vi "TPM with correction version 10-3-compare-1 scale factor_descan_20191023.vi"() -> ()   [LabVIEW 2018]
uses:
  Casao LabVIEW SDK 1.0.5/Haso/Data Haso/Wavefront parameters.ctl
  Casao LabVIEW SDK 1.0.5/Casao/Casao/Loop prefs.ctl
  Casao LabVIEW SDK 1.0.5/Haso/Data Haso/DataHaso.ctl
  <vilib>/Utility/file.llb/Read From Spreadsheet File (DBL).vi
  <vilib>/Utility/file.llb/Write To Spreadsheet File (DBL).vi
panel:
  out "error out 4":errorcluster
  out "error out 3":errorcluster
  out "error out 2":errorcluster
  out "error out":errorcluster
  in  "Descan  Rescan":bool
  in  "Camera              WF sensor":bool
  in  "Scale factor":dbl=1.0
  out "output path":path
  out "Model Coefficients (µm) after":sgl[](array[numeric])
  out "Model Coefficients (µm) before":sgl[](array[numeric])
  in  "stop":bool
  out "Slice now":dbl
  in  "Iteration #":u16(ring)=1 items=["1"=1, "2"=2, "3"=3, "4"=4, "5"=5]
  in  "AoExp Time":dbl(ring)=0.5 items=["0.2s"=0.2, "0.5s"=0.5, "1.0s"=1.0, "1.5s"=1.5]
  out "after correction":T1
  in  "Filter y tilt":bool=TRUE
  in  "Filter x tilt":bool=TRUE
  in  "Curvature filter":bool=TRUE
  out "PV":dbl
  out "RMS":dbl
  in  "Matrix path":path=path "D:/SystemAlignment/20191015_PathCheck_WFSalign/commandMatrix.aomc"
  in  "Offset path":path=path "D:/Data/100nm correction.dat"
  out "Camera image":u32[][](graph)
  out "RMS":dbl
  out "PV":dbl
  out "before correction":T1
  in  "Curvature filter":bool=TRUE
  in  "Filter y tilt":bool=TRUE
  in  "Filter x tilt":bool=TRUE
  out "after correction":dbl[][](graph) caption="Wavefront"
  out "before correction":dbl[][](graph) caption="Wavefront"
  in  "ImExp Time (s)":dbl(ring)=0.5 items=["0.2"=0.2, "0.5"=0.5, "1.0"=1.0, "4.0"=4.0, "8.0"=8.0]
  in  "Step size(um)":dbl
  in  "Laser Power%(0-100)":dbl=50.0
  in  "Slices #":dbl=2.0
  in  "Average Frame #":dbl=2.0
  in  "Correction":bool
  # "OFF"
  # "ON"
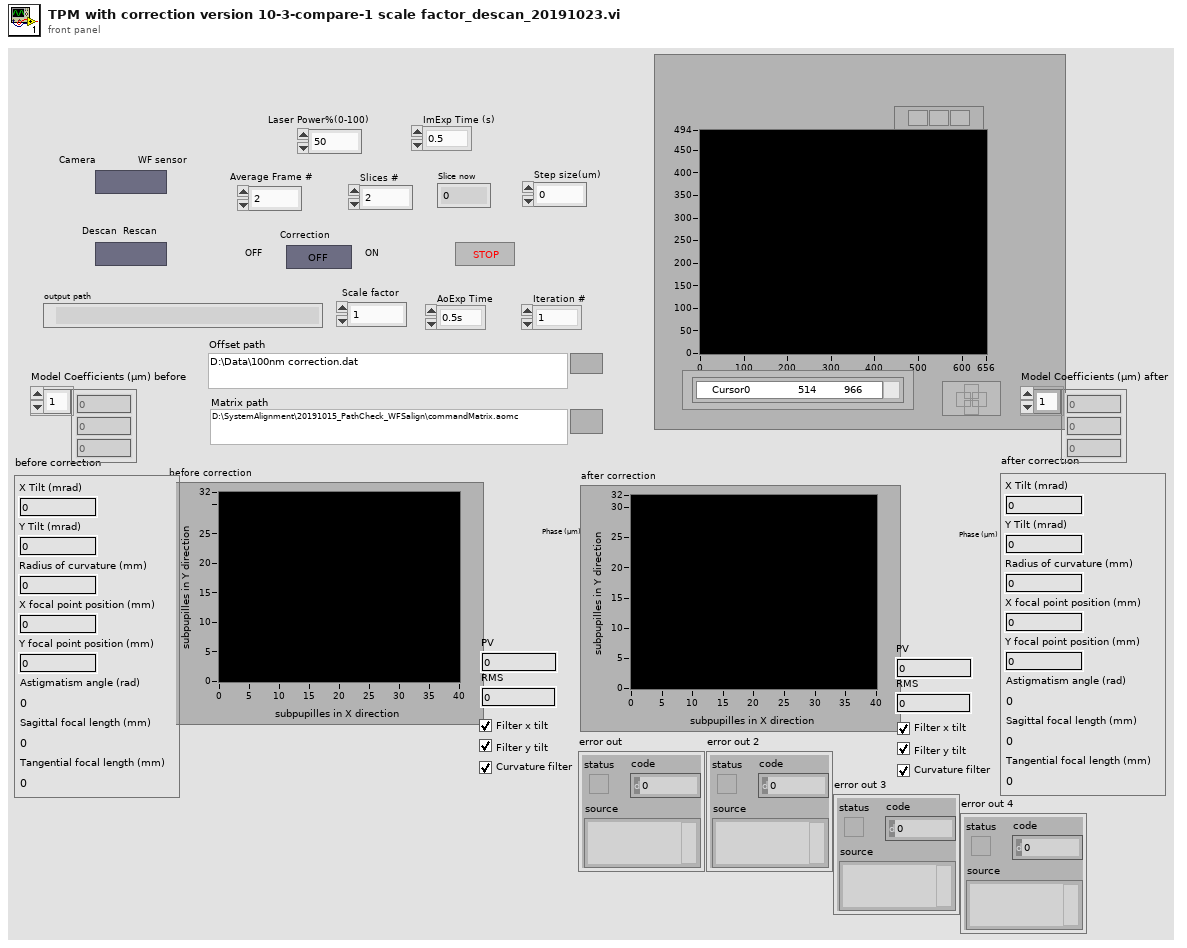
[diagram p1: front panel]
types:
  T1 = typedef "Wavefront parameters.ctl" = cluster{"X Tilt (mrad)":sgl, "Y Tilt (mrad)":sgl, "Radius of curvature (mm)":sgl, "X focal point position (mm)":sgl, "Y focal point position (mm)":sgl, "Astigmatism angle (rad)":sgl, "Sagittal focal length (mm)":sgl, "Tangential focal length (mm)":sgl}
  T2 = typedef "Loop prefs.ctl" = cluster{"Filter tilt on measurement (closed loop)":bool, "Correction gain (closed loop)":sgl, "Limit of subapertures off in CGP (%)":sgl, "Limit of saturated actuators (%)":sgl}
  T3 = cluster{"Filtre tilt X":bool, "Filtre tilt Y":bool, "Filtre courbure":bool}
  T4 = typedef "DataHaso.ctl" = i32
  T5 = cluster{"Measurement":T4, "Target":T4, "Manual target":T4}
  T6 = cluster{"Target for tilt":T4, "Target for focus":T4, "Target for all other aberrations":T4}
  T7 = typedef "Camera.ctl" = i32
  T8 = typedef "PhaseModul.ctl" = i32
  T9 = typedef "Haso.ctl" = i32
  T10 = typedef "Casao.ctl" = i32
  T11 = typedef "Image Compat.ctl" = cluster{"Signed/unsigned":bool, "Number of bits":T12, "Internal object id":i32, "Internal data id":i32}
  T12 = typedef "Data alignment enum.ctl" = enum16{"8", "16", "32"}
  T13 = typedef "Reconstruction prefs.ctl" = cluster{"Reconstruction type":enum16{"Modal", "Zonal"}, "Polynomial type":enum16{"Zernike", "Legendre"}, "Modal reconstruction prefs":T14, "Zonal reconstruction prefs":T17}
  T14 = typedef "Modal reconstruction prefs.ctl" = cluster{"Number of coefficients":u32, "Filtered coefficients":u32[], "RMS Zernike normalization":bool, "Matrix inversion method":u16, "Add zonal residual to modal fit ":bool, "Detection prefs":T15}
  T15 = typedef "PupilDetectionPrefs.ctl" = cluster{"Automatic pupil detection":bool, "Central occultation pupil":bool, "Semi-automatic pupil detection (find radius)":bool, "Semi-automatic pupil detection (find center)":bool, "Automatic pupil detection mode":enum16{"Contained", "Containing"}, "Start coordinates":cluster{"Pupil center (Zernike)":T16, "Pupil radius (Zernike)":sgl, "Pupil center (Legendre)":T16, "Pupil halfsize (Legendre)":T16}}
  T16 = typedef "Point2Df.ctl" = cluster{"X":sgl, "Y":sgl}
  T17 = typedef "Zonal reconstruction prefs.ctl" = cluster{"Number of weak iterations":u16, "Number of max iterations":u32, "Residual limit":sgl}
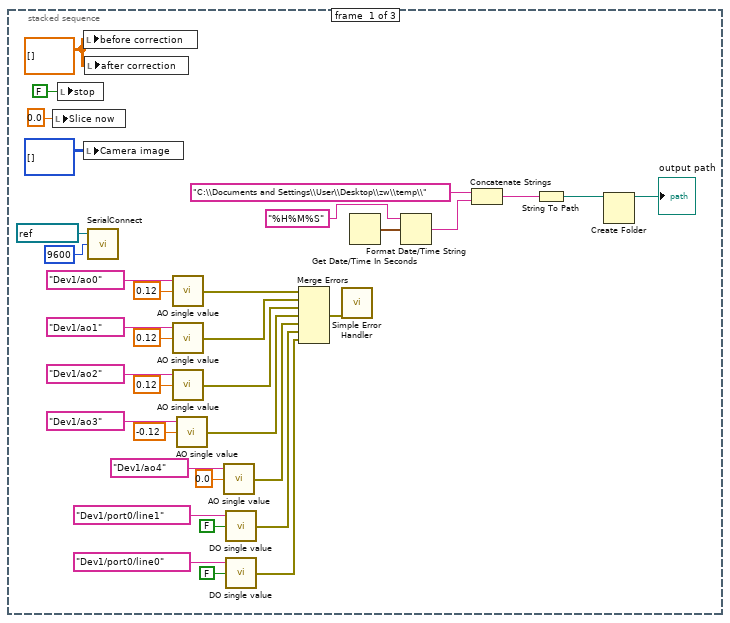
[diagram p2: hidden frame]
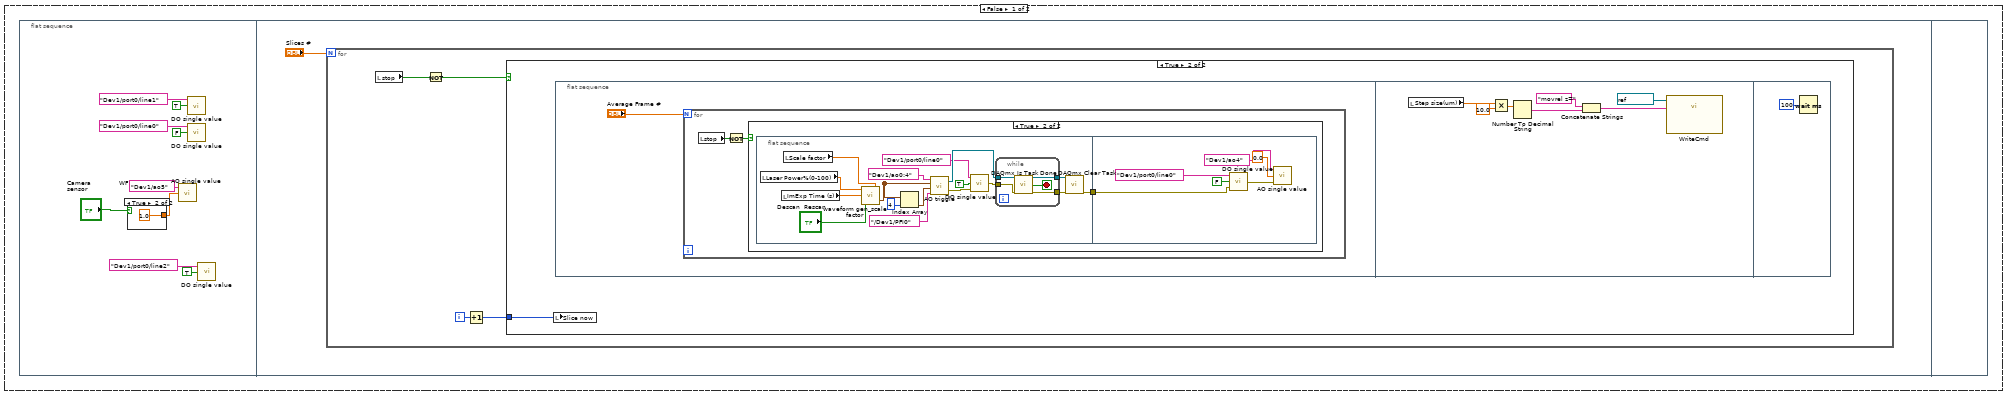
[diagram p3: hidden frame]
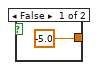
[diagram p4: hidden frame]
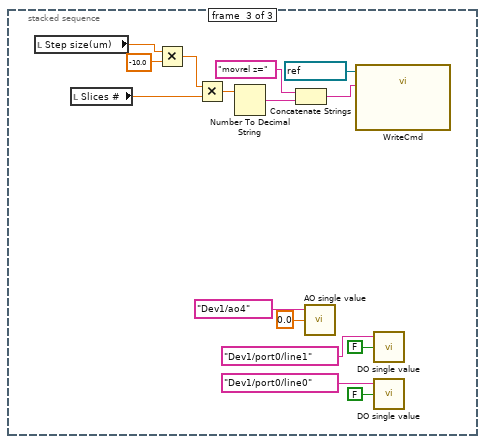
[diagram p12: hidden frame]
diagram:
  n1 = stacked-sequence {
    frame #0 {
      w34 = dbl[][] [] ("before correction")
      n2 = local write "Slice now"(0.0 ("Slice now")) -> ()
      n3 = local write "stop"(FALSE ("stop")) -> ()
      n4 = local write "before correction"(w34) -> ()
      n5 = local write "Camera image"(u32[][] [] ("Camera image")) -> ()
      n6 = local write "after correction"(w34) -> ()
      n7 = call "SerialConnect.vi"("baud rate (9600)"=u32 9600, "VISA resource name"=refnum<visa-resource-name> "COM1") -> ()  [unwired: 1 in, 3 out]
      n8 = call "AO single value.vi"("data"=0.12, "physical channels"=tag "Dev1/ao0") -> ("error out"=w17:errorcluster)  [unwired: 1 in]
      n9 = call "AO single value.vi"("data"=0.12, "physical channels"=tag "Dev1/ao1") -> ("error out"=w16:errorcluster)  [unwired: 1 in]
      n10 = call "AO single value.vi"("data"=0.12, "physical channels"=tag "Dev1/ao2") -> ("error out"=w15:errorcluster)  [unwired: 1 in]
      n11 = call "AO single value.vi"("data"=-0.12, "physical channels"=tag "Dev1/ao3") -> ("error out"=w14:errorcluster)  [unwired: 1 in]
      n12 = call "AO single value.vi"("data"=0.0, "physical channels"=tag "Dev1/ao4") -> ("error out"=w13:errorcluster)  [unwired: 1 in]
      n13 = call "DO single value.vi"("data"=FALSE, "lines"=tag "Dev1/port0/line1") -> ("error out"=w12:errorcluster)  [unwired: 1 in]
      n14 = call "DO single value.vi"("data"=FALSE, "lines"=tag "Dev1/port0/line0") -> ("error out"=w10:errorcluster)  [unwired: 1 in]
      n15 = Merge Errors(w17, w16, w15, w14, w13, w12, w10) -> (w11:errorcluster)
      n16 = call <vilib>:"Simple Error Handler.vi"("error in (no error)"=w11) -> ()  [unwired: 4 in, 5 out]
      n17 = Get Date/Time In Seconds() -> (seconds since 1Jan1904=w7:timestamp)
      n18 = Format Date/Time String(time format string (%c)="%H%M%S", seconds (now)=w7) -> (date/time string=w4:string)  [unwired: 1 in]
      n19 = Concatenate Strings("C:\\Documents and Settings\\User\\Desktop\\zw\\temp\\" ("string"), w4) -> (w3:string)
      n20 = String To Path(string=w3) -> (path=w2:path)
      n21 = Create Folder(path (use dialog)=w2) -> (created path=→"output path":path)  [unwired: 2 in, 2 out]
    }
    frame #1 {
      n22 = case shown="True" "Correction" {
        frame False {
          n23 = flat-sequence {
            frame #0 {
              n24 = case shown="True" "Camera              WF sensor" {
                tunnel: [-5.0 ("data") 1.0 ("data")] -> w40
                frame False {
                }
                frame True {
                }
              }
              n25 = call "AO single value.vi"("data"=w40, "physical channels"=tag "Dev1/ao5") -> ()  [unwired: 1 in, 1 out]
              n26 = call "DO single value.vi"("data"=TRUE, "lines"=tag "Dev1/port0/line1") -> ()  [unwired: 1 in, 1 out]
              n27 = call "DO single value.vi"("data"=FALSE, "lines"=tag "Dev1/port0/line0") -> ()  [unwired: 1 in, 1 out]
              n28 = call "DO single value.vi"("data"=TRUE, "lines"=tag "Dev1/port0/line2") -> ()  [unwired: 1 in, 1 out]
            }
            frame #1 {
              n29 = for {
                N: "Slices #" -> [_]
                i -> [w52]
                n30 = local read "stop"() -> (w50:bool)
                n31 = Not(x=w50) -> (.not. x?=w49:bool)
                n32 = Increment(x=w52) -> (x+1=w51:i32)
                n33 = case shown="True" w49 {
                  tunnel: w51 -> [_ w53]
                  frame False {
                  }
                  frame True {
                    n34 = local write "Slice now"(w53) -> ()
                    n35 = flat-sequence {
                      frame #0 {
                        n36 = for {
                          N: "Average Frame #" -> [_]
                          n37 = local read "stop"() -> (w55:bool)
                          n38 = Not(x=w55) -> (.not. x?=w56:bool)
                          n39 = case shown="True" w56 {
                            frame False {
                            }
                            frame True {
                              n40 = flat-sequence {
                                tunnel: [w63] -> w57
                                tunnel: w57 -> [w81]
                                frame #0 {
                                n41 = local read "Laser Power%(0-100)"() -> (w60:dbl)
                                n42 = local read "ImExp Time (s)"() -> (w61:dbl)
                                n43 = local read "Scale factor"() -> (w59:dbl)
                                n44 = call "waveform gen_scale factor.vi"("Scale factor"=w59, "Boolean"="Descan  Rescan", "Exposure Time (s)"=w61, "Laser Power%(0-100)"=w60) -> ("waveform"=w62:waveform(dbl)[])
                                n45 = Index Array(array=w62, index=4) -> (element=w71:waveform(dbl))
                                n46 = call "AO triggle.vi"("physical channels"=tag "Dev1/ao0:4", "data"=w62, "waveform"=w71, "trig source"=tag "/Dev1/PFI0") -> ("task out"=w68:refnum<k21>, "error out"=w65:errorcluster)  [unwired: 1 in]
                                n47 = call "DO single value.vi"("error in"=w65, "data"=TRUE, "lines"=tag "Dev1/port0/line0") -> ("error out"=w64:errorcluster)
                                n48 = while {
                                tunnel: [w79] -> w74
                                tunnel: [w78] -> w73
                                tunnel: w68 -> [w76]
                                tunnel: w64 -> [w75]
                                stop <- w77 stop-if-true
                                n49 = call <vilib>:"DAQmx Is Task Done.vi"("task/channels in"=w76, "error in"=w75) -> ("task out"=w79:refnum<k21>, "task done?"=w77:bool, "error out"=w78:errorcluster)  [unwired: 11 in]
                                }
                                n50 = call <vilib>:"DAQmx Clear Task.vi"("task in"=w74, "error in"=w73) -> ("error out"=w63:errorcluster)  [unwired: 13 in]
                                }
                                frame #1 {
                                n51 = call "DO single value.vi"("error in"=w81, "data"=FALSE, "lines"=tag "Dev1/port0/line0") -> ("error out"=w80:errorcluster)
                                n52 = call "AO single value.vi"("error in"=w80, "data"=0.0, "physical channels"=tag "Dev1/ao4") -> ()  [unwired: 1 out]
                                }
                              }
                            }
                          }
                        }
                      }
                      frame #1 {
                        n53 = local read "Step size(um)"() -> (w86:dbl)
                        n54 = Multiply(x=w86, y=10.0) -> (x*y=w88:dbl)
                        n55 = Number To Decimal String(number=w88) -> (decimal integer string=w91:string)  [unwired: 1 in]
                        n56 = Concatenate Strings("movrel z=", w91) -> (w90:string)
                        n57 = call "WriteCmd.vi"("Command"=w90, "VISA resource name"=refnum<visa-resource-name> "COM1") -> ()  [unwired: 1 in, 1 out]
                      }
                      frame #2 {
                        n58 = Wait (ms)(milliseconds to wait=u32 100) -> ()  [unwired: 1 out]
                      }
                    }
                  }
                }
              }
            }
            frame #2 {
            }
          }
        }
        frame True {
          n59 = flat-sequence {
            tunnel: [w102] -> w101
            tunnel: [w111] -> w100
            tunnel: [w110] -> w99
            tunnel: [w102] -> w98
            tunnel: [w109] -> w97
            tunnel: [w108] -> w95
            tunnel: [w103] -> w94
            tunnel: w101 -> [w128]
            tunnel: w100 -> [w127]
            tunnel: w99 -> [w126]
            tunnel: w98 -> [w122]
            tunnel: w97 -> [w120]
            tunnel: [w125] -> w96
            tunnel: w95 -> [w124]
            tunnel: w94 -> [w118]
            tunnel: w96 -> [w655]
            frame #0 {
              n60 = call "AO single value.vi"("data"=0.0, "physical channels"=tag "Dev1/ao4") -> ()  [unwired: 1 in, 1 out]
              n61 = local read "AoExp Time"() -> (w112:dbl)
              n62 = call-poly <vilib>:"Read From Spreadsheet File.vi"("format (%.3f)"="%.8f", "file path (dialog if empty)"="Offset path") -> ("first row"=w103:dbl[])  [unwired: 5 in, 4 out]
              n63 = call "DO single value.vi"("data"=TRUE, "lines"=tag "Dev1/port0/line1") -> ()  [unwired: 1 in, 1 out]
              n64 = call "DO single value.vi"("data"=FALSE, "lines"=tag "Dev1/port0/line0") -> ()  [unwired: 1 in, 1 out]
              n65 = call "AO init.vi"("Exposure duration specified (s)"=w112, "Commands in"=w103, "Matrix path"="Matrix path") -> ("error out"=w102:errorcluster, "Camera"=w111:T7, "Mirror"=w108:T8, "Haso"=w110:T9, "Casao"=w109:T10)  [unwired: 3 in, 1 out]
              "error out" <- w102
            }
            frame #1 {
              n66 = local read "Slices #"() -> (w129:dbl)
              n67 = call "Casao Set Preferences.vi"("error in (no error)"=w122, "Loop preferences"=T2 {"Filter tilt on measurement (closed loop)"=FALSE, "Correction gain (closed loop)"=0.75, "Limit of subapertures off in CGP (%)"=0.0, "Limit of saturated actuators (%)"=0.0}, "Casao"=w120) -> ("error out"=w121:errorcluster, "Casao (dup)"=w119:T10)  [unwired: 3 in]
              n68 = for {
                N: w129 -> [_]
                tunnel: w128 -> [w145]
                tunnel: w127 -> [w144]
                tunnel: w126 -> [w143]
                tunnel: w121 -> [w131]
                tunnel: [w142] -> w125
                tunnel: w124 -> [w133]
                tunnel: w119 -> [w141]
                tunnel: w118 -> [w134]
                i -> [w137]
                n69 = local read "stop"() -> (w139:bool)
                n70 = call "PhaseModul apply command.vi"("error in (no error)"=w131, "Commands in"=w134, "Mirror"=w133) -> ("error out"=w130:errorcluster, "Mirror (dup)"=w132:T8)  [unwired: 2 in, 1 out]
                n71 = Increment(x=w137) -> (x+1=w140:i32)
                n72 = local write "Slice now"(w140) -> ()
                n73 = Not(x=w139) -> (.not. x?=w138:bool)
                n74 = case shown="True" w138 {
                  tunnel: w145 -> [_ w180]
                  tunnel: w144 -> [_ w179]
                  tunnel: w143 -> [_ w178]
                  tunnel: w130 -> [_ w177]
                  tunnel: [w146 w174] -> w142
                  tunnel: w132 -> [_ w176]
                  tunnel: w141 -> [w146 w175]
                  frame False {
                  }
                  frame True {
                    n75 = flat-sequence {
                      tunnel: w175 -> [w185]
                      tunnel: w176 -> [w186]
                      tunnel: w177 -> [w187]
                      tunnel: w178 -> [w188]
                      tunnel: w179 -> [w189]
                      tunnel: w180 -> [w190]
                      tunnel: [w190] -> w152
                      tunnel: [w189] -> w151
                      tunnel: [w188] -> w150
                      tunnel: [w187] -> w149
                      tunnel: [w186] -> w148
                      tunnel: [w185] -> w147
                      tunnel: [w226] -> w173
                      tunnel: [w225] -> w172
                      tunnel: [w224] -> w171
                      tunnel: [w219] -> w170
                      tunnel: [w220] -> w169
                      tunnel: [w221] -> w168
                      tunnel: w152 -> [w226]
                      tunnel: w151 -> [w225]
                      tunnel: w150 -> [w224]
                      tunnel: w149 -> [w220]
                      tunnel: w148 -> [w221]
                      tunnel: w147 -> [w219]
                      tunnel: w173 -> [w268]
                      tunnel: w172 -> [w267]
                      tunnel: w171 -> [w266]
                      tunnel: w170 -> [w265]
                      tunnel: w169 -> [w264]
                      tunnel: [w244] -> w167
                      tunnel: [w243] -> w166
                      tunnel: [w239] -> w165
                      tunnel: [w237] -> w164
                      tunnel: [w235] -> w163
                      tunnel: w168 -> [w230]
                      tunnel: [w229] -> w162
                      tunnel: [w227] -> w161
                      tunnel: w167 -> [w410]
                      tunnel: w166 -> [w409]
                      tunnel: w165 -> [w407]
                      tunnel: w164 -> [w406]
                      tunnel: w163 -> [w405]
                      tunnel: [w404] -> w160
                      tunnel: w162 -> [w403]
                      tunnel: [w402] -> w159
                      tunnel: [w401] -> w158
                      tunnel: [w400] -> w157
                      tunnel: [w399] -> w156
                      tunnel: [w398] -> w155
                      tunnel: w161 -> [w397]
                      tunnel: [w397] -> w154
                      tunnel: w160 -> [w617]
                      tunnel: [w617] -> w153
                      tunnel: w159 -> [w607]
                      tunnel: w158 -> [w606]
                      tunnel: w157 -> [w605]
                      tunnel: w156 -> [w595]
                      tunnel: w155 -> [w596]
                      tunnel: w154 -> [w594]
                      tunnel: w153 -> [w618]
                      tunnel: [w618] -> w174
                      frame #0 {
                        n76 = local read "Average Frame #"() -> (w184:dbl)
                        n77 = Wait (ms)(milliseconds to wait=u32 100) -> ()  [unwired: 1 out]
                        n78 = call "AO single value.vi"("data"=-5.0, "physical channels"=tag "Dev1/ao5") -> ()  [unwired: 1 in, 1 out]
                        n79 = for {
                          N: w184 -> [_]
                          n80 = local read "stop"() -> (w191:bool)
                          n81 = Not(x=w191) -> (.not. x?=w192:bool)
                          n82 = case shown="True" w192 {
                            frame False {
                            }
                            frame True {
                              n83 = flat-sequence {
                                frame #0 {
                                n84 = local read "Laser Power%(0-100)"() -> (w194:dbl)
                                n85 = local read "ImExp Time (s)"() -> (w195:dbl)
                                n86 = local read "Scale factor"() -> (w193:dbl)
                                n87 = call "waveform gen_scale factor.vi"("Scale factor"=w193, "Boolean"=TRUE, "Exposure Time (s)"=w195, "Laser Power%(0-100)"=w194) -> ("waveform"=w197:waveform(dbl)[])
                                n88 = Index Array(array=w197, index=4) -> (element=w205:waveform(dbl))
                                n89 = call "AO triggle.vi"("physical channels"=tag "Dev1/ao0:4", "data"=w197, "waveform"=w205, "trig source"=tag "/Dev1/PFI0") -> ("task out"=w202:refnum<k21>, "error out"=w199:errorcluster)  [unwired: 1 in]
                                n90 = call "DO single value.vi"("error in"=w199, "data"=TRUE, "lines"=tag "Dev1/port0/line0") -> ("error out"=w198:errorcluster)
                                n91 = while {
                                tunnel: [w213] -> w208
                                tunnel: [w212] -> w207
                                tunnel: w202 -> [w210]
                                tunnel: w198 -> [w209]
                                stop <- w211 stop-if-true
                                n92 = call <vilib>:"DAQmx Is Task Done.vi"("task/channels in"=w210, "error in"=w209) -> ("task out"=w213:refnum<k21>, "task done?"=w211:bool, "error out"=w212:errorcluster)  [unwired: 11 in]
                                }
                                n93 = call <vilib>:"DAQmx Clear Task.vi"("task in"=w208, "error in"=w207) -> ()  [unwired: 13 in, 1 out]
                                }
                                frame #1 {
                                n94 = call "AO single value.vi"("data"=0.0, "physical channels"=tag "Dev1/ao4") -> ()  [unwired: 1 in, 1 out]
                                n95 = call "DO single value.vi"("data"=FALSE, "lines"=tag "Dev1/port0/line0") -> ()  [unwired: 1 in, 1 out]
                                }
                              }
                            }
                          }
                        }
                      }
                      frame #1 {
                        n96 = call "AO single value.vi"("data"=1.0, "physical channels"=tag "Dev1/ao5") -> ("error out"=→"error out 4":errorcluster)  [unwired: 1 in]
                      }
                      frame #2 {
                        n97 = flat-sequence {
                          tunnel: [w277] -> w263
                          tunnel: [w276] -> w262
                          tunnel: [w275] -> w261
                          tunnel: [w274] -> w260
                          tunnel: [w273] -> w259
                          tunnel: w266 -> [w275]
                          tunnel: w267 -> [w276]
                          tunnel: w268 -> [w277]
                          tunnel: [w272] -> w258
                          tunnel: w265 -> [w272]
                          tunnel: [w271] -> w257
                          tunnel: w264 -> [w271]
                          tunnel: [w270] -> w231
                          tunnel: w230 -> [w270]
                          tunnel: w263 -> [w293]
                          tunnel: w262 -> [w294]
                          tunnel: w261 -> [w295]
                          tunnel: [w295] -> w256
                          tunnel: [w292] -> w255
                          tunnel: [w286] -> w254
                          tunnel: [w291] -> w253
                          tunnel: w260 -> [w291]
                          tunnel: [w290] -> w252
                          tunnel: w259 -> [w290]
                          tunnel: [w289] -> w251
                          tunnel: w258 -> [w289]
                          tunnel: [w288] -> w250
                          tunnel: w257 -> [w288]
                          tunnel: [w287] -> w232
                          tunnel: w231 -> [w287]
                          tunnel: w256 -> [w307]
                          tunnel: [w307] -> w247
                          tunnel: [w306] -> w248
                          tunnel: w255 -> [w306]
                          tunnel: [w305] -> w249
                          tunnel: w254 -> [w305]
                          tunnel: w253 -> [w300]
                          tunnel: w252 -> [w299]
                          tunnel: [w298] -> w246
                          tunnel: w251 -> [w298]
                          tunnel: [w297] -> w245
                          tunnel: w250 -> [w297]
                          tunnel: [w296] -> w233
                          tunnel: w232 -> [w296]
                          tunnel: w249 -> [w389]
                          tunnel: w248 -> [w350]
                          tunnel: w247 -> [w351]
                          tunnel: w246 -> [w375]
                          tunnel: w245 -> [w374]
                          tunnel: [w354] -> w242
                          tunnel: [w353] -> w241
                          tunnel: [w352] -> w240
                          tunnel: [w351] -> w238
                          tunnel: [w350] -> w236
                          tunnel: [w349] -> w234
                          tunnel: w233 -> [w348]
                          tunnel: [w348] -> w228
                          tunnel: [w322] -> w227
                          tunnel: [w395] -> w243
                          tunnel: [w396] -> w244
                          tunnel: w242 -> [w396]
                          tunnel: w241 -> [w395]
                          tunnel: w240 -> [w394]
                          tunnel: [w393] -> w239
                          tunnel: w238 -> [w393]
                          tunnel: [w392] -> w237
                          tunnel: w236 -> [w392]
                          tunnel: [w391] -> w235
                          tunnel: w234 -> [w391]
                          tunnel: [w390] -> w229
                          tunnel: w228 -> [w390]
                          frame #0 {
                            n98 = local read "Laser Power%(0-100)"() -> (w283:dbl)
                            n99 = local read "AoExp Time"() -> (w282:dbl)
                            n100 = local read "Scale factor"() -> (w269:dbl)
                            n101 = call "waveform gen_scale factor.vi"("Scale factor"=w269, "Boolean"=FALSE, "Exposure Time (s)"=w282, "Laser Power%(0-100)"=w283) -> ("waveform"=w281:waveform(dbl)[])
                            n102 = Index Array(array=w281, index=4) -> (element=w280:waveform(dbl))
                            n103 = call "AO triggle.vi"("physical channels"=tag "Dev1/ao0:4", "data"=w281, "waveform"=w280, "trig source"=tag "/Dev1/PFI0") -> ("task out"=w274:refnum<k21>, "error out"=w273:errorcluster)  [unwired: 1 in]
                          }
                          frame #1 {
                            n104 = call "Camera Start.vi"("error in (no error)"=w293, "camera"=w294) -> ("error out"=w286:errorcluster, "camera (dup)"=w292:T7)  [unwired: 4 in]
                            "error out 2" <- w286
                          }
                          frame #2 {
                            n105 = while {
                              tunnel: [w312] -> w302
                              tunnel: [w311] -> w301
                              tunnel: w300 -> [w309]
                              tunnel: w299 -> [w308]
                              stop <- w310 stop-if-true
                              n106 = call <vilib>:"DAQmx Is Task Done.vi"("task/channels in"=w309, "error in"=w308) -> ("task out"=w312:refnum<k21>, "task done?"=w310:bool, "error out"=w311:errorcluster)  [unwired: 11 in]
                            }
                            n107 = call "DO single value.vi"("data"=TRUE, "lines"=tag "Dev1/port0/line0") -> ()  [unwired: 1 in, 1 out]
                            n108 = call <vilib>:"DAQmx Clear Task.vi"("task in"=w302, "error in"=w301) -> ()  [unwired: 13 in, 1 out]
                          }
                          frame #3 {
                            n109 = call "Camera Get image.vi"("error in (no error)"=w389, "camera"=w350) -> ("error out"=w371:errorcluster, "Image"=w372:T11, "camera (dup)"=w373:T7)  [unwired: 3 in]
                            n110 = call "Camera Stop.vi"("error in (no error)"=w371, "camera"=w373) -> ()  [unwired: 4 in, 2 out]
                            n111 = call "Image get data.vi"("error in (no error)"=w371, "Image Compat"=w372) -> ("error out"=w313:errorcluster, "Array"=w370:u32[][], "Image Compat (dup)"=w361:T11)  [unwired: 3 in]
                            "error out 3" <- w313
                            n112 = call "AO single value.vi"("data"=0.0, "physical channels"=tag "Dev1/ao4") -> ()  [unwired: 1 in, 1 out]
                            n113 = local write "Camera image"(w370) -> ()
                            n114 = call "Haso compute slopes.vi"("error in (no error)"=w313, "Image Compat"=w361, "Haso"=w351) -> ("error out"=w320:errorcluster, "Data Haso"=w324:T4)  [unwired: 1 in, 2 out]
                            n115 = call "DO single value.vi"("data"=FALSE, "lines"=tag "Dev1/port0/line0") -> ()  [unwired: 1 in, 1 out]
                            n116 = call "DataHaso ctor copie.vi"("error in (no error)"=w320, "DataHaso"=w324) -> ("error out"=w319:errorcluster, "new DataHaso"=w322:T4, "DataHaso (dup)"=w321:T4)  [unwired: 3 in]
                            n117 = call "DataHaso get reconstruction prefs.vi"("error in (no error)"=w319, "Data Haso"=w321) -> ("error out"=w335:errorcluster, "Reconstruction Preferences"=w331:T13, "Data Haso (dup)"=w334:T4)  [unwired: 3 in]
                            n118 = Bundle By Name(cluster=w331, "Reconstruction type"=enum16{"Modal", "Zonal"}."Modal", "Polynomial type"=enum16{"Zernike", "Legendre"}."Zernike", "Modal reconstruction prefs.Number of coefficients"=u32 32) -> (w330:T13)
                            n119 = call "DataHaso set reconstruction prefs.vi"("error in (no error)"=w335, "Reconstruction Preferences"=w330, "Data Haso"=w334) -> ("error out"=w332:errorcluster, "Data Haso (dup)"=w333:T4)  [unwired: 3 in]
                            n120 = call "DataHaso get modal coefficients.vi"("error in (no error)"=w332, "Data Haso"=w333) -> ("error out"=w325:errorcluster, "Coefficients (µm)"=w336:sgl[], "Data Haso (dup)"=w326:T4)  [unwired: 3 in]
                            "Model Coefficients (µm) before" <- w336
                            n121 = Bundle By Name(cluster=T3 {"Filtre tilt X"=FALSE, "Filtre tilt Y"=FALSE, "Filtre courbure"=FALSE} ("Filtre"), "Filtre tilt X"="Filter x tilt", "Filtre tilt Y"="Filter y tilt", "Filtre courbure"="Curvature filter") -> (w356:T3)
                            n122 = call "DataHaso parameters.vi"("error in (no error)"=w325, "Data Haso"=w326) -> ("error out"=w368:errorcluster, "Parameters"=w344:T1, "Data Haso (dup)"=w369:T4)  [unwired: 3 in]
                            "before correction" <- w344
                            n123 = control-ref of="before correction"() -> (w355:refnum<vi>)
                            n124 = Cluster To Array(cluster=w344) -> (array=w345:sgl[])
                            n125 = call "DataHaso filter tilt or curvature.vi"("error in (no error)"=w368, "Filter (default: all true)"=w356, "Data Haso"=w369) -> ("error out"=w366:errorcluster, "Data Haso (dup)"=w367:T4)  [unwired: 3 in]
                            n126 = local read "Slice now"() -> (w338:dbl)
                            n127 = call "DataHaso phase.vi"("error in (no error)"=w366, "Data Haso"=w367) -> ("error out"=w364:errorcluster, "Phase (µm)"=w365:i32, "Data Haso (dup)"=w323:T4)  [unwired: 3 in]
                            n128 = Number To Decimal String(number=w338) -> (decimal integer string=w340:string)  [unwired: 1 in]
                            n129 = call "Formatter Intensity Graph.vi"("error in (no error)"=w364, "Intensity Graph"=w355, "Surface with pupil"=w365) -> ("error out"=w362:errorcluster, "Surface with pupil (dup)"=w363:i32)  [unwired: 2 in, 1 out]
                            n130 = call "Surface with pupil get stats.vi"("error in (no error)"=w362, "Surface Avec Pupille"=w363) -> ("error out"=w349:errorcluster, "PV"=w347:sgl, "RMS"=w346:dbl)  [unwired: 2 in, 1 out]
                            "PV" <- w347
                            "RMS" <- w346
                            n131 = local read "output path"() -> (w316:path)
                            n132 = Concatenate Strings("before_slice", w340, ".dat") -> (w315:string)
                            n133 = Build Path(base path=w316, name or relative path=w315) -> (appended path=w314:path)
                            n134 = Build Array (concatenate)(w347, w346, w345, w336) -> (w343:dbl[])
                            n135 = Merge Errors(w349, w374) -> (w384:errorcluster)
                            n136 = Bundle By Name(cluster=T6 {"Target for tilt"=0, "Target for focus"=0, "Target for all other aberrations"=0} ("References"), "Target for tilt"=w322, "Target for focus"=w322) -> (w387:T6)
                            n137 = call "DataHaso ctor copie.vi"("error in (no error)"=w384, "DataHaso"=w323) -> ("error out"=w386:errorcluster, "new DataHaso"=w385:T4)  [unwired: 3 in, 1 out]
                            n138 = call-poly <vilib>:"Write To Spreadsheet File.vi"("transpose? (no:F)"=TRUE, "format (%.3f)"="%.6f", "1D data"=w343, "file path (dialog if empty)"=w314) -> ()  [unwired: 4 in, 1 out]
                            n139 = call "Casao Compute target.vi"("error in (no error)"=w386, "Targets"=w387, "DataHaso"=w385, "Casao"=w375) -> ("error out"=w382:errorcluster, "DataHaso (dup)"=w352:T4, "Casao (dup)"=w383:T10)  [unwired: 1 out]
                            n140 = Bundle By Name(cluster=T5 {"Measurement"=0, "Target"=0, "Manual target"=0} ("Slopes"), "Measurement"=w323, "Target"=w352) -> (w381:T5)
                            n141 = call "Casao get correction commands.vi"("Casao"=w383, "Slopes"=w381, "error in (no error)"=w382) -> ("Casao (dup)"=w354:T10, "Commands"=w378:sgl[], "error out"=w379:errorcluster)  [unwired: 2 in, 2 out]
                            n142 = call "PhaseModul apply command.vi"("error in (no error)"=w379, "Commands in"=w378, "Mirror"=w348) -> ("error out"=w353:errorcluster)  [unwired: 2 in, 2 out]
                          }
                          frame #4 {
                            n143 = call "DataHaso dtor.vi"("Data Haso"=w394) -> ()  [unwired: 6 in, 1 out]
                          }
                        }
                      }
                      frame #3 {
                        n144 = for {
                          N: "Iteration #" -> [_]
                          tunnel: w410 -> [w439]
                          tunnel: w409 -> [w438]
                          tunnel: w407 -> [w437]
                          tunnel: w406 -> [w436]
                          tunnel: w405 -> [w435]
                          tunnel: [w433] -> w404
                          tunnel: w403 -> [w428]
                          tunnel: [w427] -> w402
                          tunnel: [w425] -> w401
                          tunnel: [w423] -> w400
                          tunnel: [w421] -> w399
                          tunnel: [w418] -> w398
                          tunnel: w397 -> [w417]
                          i -> [w416]
                          n145 = Increment(x=w416) -> (x+1=w415:i32)
                          n146 = flat-sequence {
                            tunnel: [w464] -> w458
                            tunnel: [w465] -> w457
                            tunnel: [w466] -> w456
                            tunnel: [w470] -> w455
                            tunnel: [w469] -> w454
                            tunnel: [w468] -> w453
                            tunnel: [w467] -> w452
                            tunnel: w439 -> [w468]
                            tunnel: w438 -> [w467]
                            tunnel: w437 -> [w466]
                            tunnel: w436 -> [w465]
                            tunnel: w435 -> [w464]
                            tunnel: [w463] -> w429
                            tunnel: w428 -> [w463]
                            tunnel: w415 -> [w461]
                            tunnel: [w460] -> w412
                            tunnel: w458 -> [w487]
                            tunnel: w457 -> [w488]
                            tunnel: w456 -> [w489]
                            tunnel: [w489] -> w451
                            tunnel: [w486] -> w450
                            tunnel: [w485] -> w449
                            tunnel: [w484] -> w448
                            tunnel: w455 -> [w484]
                            tunnel: [w483] -> w447
                            tunnel: w454 -> [w483]
                            tunnel: [w482] -> w446
                            tunnel: w453 -> [w482]
                            tunnel: [w481] -> w445
                            tunnel: w452 -> [w481]
                            tunnel: [w480] -> w430
                            tunnel: w429 -> [w480]
                            tunnel: [w479] -> w413
                            tunnel: w412 -> [w479]
                            tunnel: w451 -> [w502]
                            tunnel: [w502] -> w442
                            tunnel: [w501] -> w443
                            tunnel: w450 -> [w501]
                            tunnel: [w500] -> w444
                            tunnel: w449 -> [w500]
                            tunnel: w448 -> [w495]
                            tunnel: w447 -> [w494]
                            tunnel: [w493] -> w441
                            tunnel: w446 -> [w493]
                            tunnel: [w492] -> w440
                            tunnel: w445 -> [w492]
                            tunnel: [w491] -> w431
                            tunnel: w430 -> [w491]
                            tunnel: [w490] -> w414
                            tunnel: w413 -> [w490]
                            tunnel: w444 -> [w570]
                            tunnel: w443 -> [w571]
                            tunnel: w442 -> [w572]
                            tunnel: w441 -> [w557]
                            tunnel: w440 -> [w556]
                            tunnel: [w536] -> w434
                            tunnel: [w535] -> w432
                            tunnel: w431 -> [w515]
                            tunnel: [w531] -> w426
                            tunnel: [w530] -> w424
                            tunnel: [w529] -> w422
                            tunnel: [w528] -> w420
                            tunnel: [w517] -> w419
                            tunnel: w417 -> [w514]
                            tunnel: w414 -> [w511]
                            tunnel: [w508] -> w411
                            tunnel: w434 -> [w584]
                            tunnel: [w583] -> w433
                            tunnel: w432 -> [w583]
                            tunnel: [w582] -> w427
                            tunnel: w426 -> [w582]
                            tunnel: [w581] -> w425
                            tunnel: w424 -> [w581]
                            tunnel: [w580] -> w423
                            tunnel: w422 -> [w580]
                            tunnel: [w576] -> w421
                            tunnel: w420 -> [w577]
                            tunnel: w419 -> [w579]
                            tunnel: [w579] -> w418
                            tunnel: w411 -> [w578]
                            frame #0 {
                              n147 = local read "Laser Power%(0-100)"() -> (w476:dbl)
                              n148 = local read "AoExp Time"() -> (w475:dbl)
                              n149 = local read "Scale factor"() -> (w459:dbl)
                              n150 = call "waveform gen_scale factor.vi"("Scale factor"=w459, "Boolean"=FALSE, "Exposure Time (s)"=w475, "Laser Power%(0-100)"=w476) -> ("waveform"=w474:waveform(dbl)[])
                              n151 = local read "Iteration #"() -> (w462:u16)
                              n152 = Index Array(array=w474, index=4) -> (element=w473:waveform(dbl))
                              n153 = Less?(x=w462, y=w461) -> (x < y?=w460:bool)
                              n154 = call "AO triggle.vi"("physical channels"=tag "Dev1/ao0:4", "data"=w474, "waveform"=w473, "trig source"=tag "/Dev1/PFI0") -> ("task out"=w470:refnum<k21>, "error out"=w469:errorcluster)  [unwired: 1 in]
                            }
                            frame #1 {
                              n155 = call "Camera Start.vi"("error in (no error)"=w487, "camera"=w488) -> ("error out"=w485:errorcluster, "camera (dup)"=w486:T7)  [unwired: 4 in]
                            }
                            frame #2 {
                              n156 = while {
                                tunnel: [w507] -> w497
                                tunnel: [w506] -> w496
                                tunnel: w495 -> [w504]
                                tunnel: w494 -> [w503]
                                stop <- w505 stop-if-true
                                n157 = call <vilib>:"DAQmx Is Task Done.vi"("task/channels in"=w504, "error in"=w503) -> ("task out"=w507:refnum<k21>, "task done?"=w505:bool, "error out"=w506:errorcluster)  [unwired: 11 in]
                              }
                              n158 = call "DO single value.vi"("data"=TRUE, "lines"=tag "Dev1/port0/line0") -> ()  [unwired: 1 in, 1 out]
                              n159 = call <vilib>:"DAQmx Clear Task.vi"("task in"=w497, "error in"=w496) -> ()  [unwired: 13 in, 1 out]
                            }
                            frame #3 {
                              n160 = call "Camera Get image.vi"("error in (no error)"=w570, "camera"=w571) -> ("error out"=w553:errorcluster, "Image"=w554:T11, "camera (dup)"=w555:T7)  [unwired: 3 in]
                              n161 = call "Camera Stop.vi"("error in (no error)"=w553, "camera"=w555) -> ()  [unwired: 4 in, 2 out]
                              n162 = call "Image get data.vi"("error in (no error)"=w553, "Image Compat"=w554) -> ("error out"=w543:errorcluster, "Array"=w552:u32[][], "Image Compat (dup)"=w542:T11)  [unwired: 3 in]
                              n163 = call "AO single value.vi"("data"=0.0, "physical channels"=tag "Dev1/ao4") -> ()  [unwired: 1 in, 1 out]
                              n164 = local write "Camera image"(w552) -> ()
                              n165 = call "Haso compute slopes.vi"("error in (no error)"=w543, "Image Compat"=w542, "Haso"=w572) -> ("error out"=w520:errorcluster, "Data Haso"=w519:T4)  [unwired: 1 in, 2 out]
                              n166 = call "DO single value.vi"("data"=FALSE, "lines"=tag "Dev1/port0/line0") -> ()  [unwired: 1 in, 1 out]
                              n167 = call "DataHaso get reconstruction prefs.vi"("error in (no error)"=w520, "Data Haso"=w519) -> ("error out"=w526:errorcluster, "Reconstruction Preferences"=w525:T13, "Data Haso (dup)"=w527:T4)  [unwired: 3 in]
                              n168 = Bundle By Name(cluster=w525, "Reconstruction type"=enum16{"Modal", "Zonal"}."Modal", "Polynomial type"=enum16{"Zernike", "Legendre"}."Zernike", "Modal reconstruction prefs.Number of coefficients"=u32 32) -> (w524:T13)
                              n169 = call "DataHaso set reconstruction prefs.vi"("error in (no error)"=w526, "Reconstruction Preferences"=w524, "Data Haso"=w527) -> ("error out"=w512:errorcluster, "Data Haso (dup)"=w513:T4)  [unwired: 3 in]
                              n170 = call "DataHaso get modal coefficients.vi"("error in (no error)"=w512, "Data Haso"=w513) -> ("error out"=w518:errorcluster, "Coefficients (µm)"=w517:sgl[], "Data Haso (dup)"=w516:T4)  [unwired: 3 in]
                              "Model Coefficients (µm) after" <- w517
                              n171 = Bundle By Name(cluster=T3 {"Filtre tilt X"=FALSE, "Filtre tilt Y"=FALSE, "Filtre courbure"=FALSE} ("Filtre"), "Filtre tilt X"="Filter x tilt", "Filtre tilt Y"="Filter y tilt", "Filtre courbure"="Curvature filter") -> (w540:T3)
                              n172 = call "DataHaso parameters.vi"("error in (no error)"=w518, "Data Haso"=w516) -> ("error out"=w550:errorcluster, "Parameters"=w529:T1, "Data Haso (dup)"=w551:T4)  [unwired: 3 in]
                              "after correction" <- w529
                              n173 = control-ref of="after correction"() -> (w534:refnum<vi>)
                              n174 = call "DataHaso filter tilt or curvature.vi"("error in (no error)"=w550, "Filter (default: all true)"=w540, "Data Haso"=w551) -> ("error out"=w548:errorcluster, "Data Haso (dup)"=w549:T4)  [unwired: 3 in]
                              n175 = call "DataHaso phase.vi"("error in (no error)"=w548, "Data Haso"=w549) -> ("error out"=w546:errorcluster, "Phase (µm)"=w547:i32, "Data Haso (dup)"=w533:T4)  [unwired: 3 in]
                              n176 = call "Formatter Intensity Graph.vi"("error in (no error)"=w546, "Intensity Graph"=w534, "Surface with pupil"=w547) -> ("error out"=w544:errorcluster, "Surface with pupil (dup)"=w545:i32)  [unwired: 2 in, 1 out]
                              n177 = call "Surface with pupil get stats.vi"("error in (no error)"=w544, "Surface Avec Pupille"=w545) -> ("error out"=w565:errorcluster, "PV"=w530:sgl, "RMS"=w531:dbl)  [unwired: 2 in, 1 out]
                              "RMS" <- w531
                              "PV" <- w530
                              n178 = Merge Errors(w565, w556) -> (w564:errorcluster)
                              n179 = Bundle By Name(cluster=T6 {"Target for tilt"=0, "Target for focus"=0, "Target for all other aberrations"=0} ("References"), "Target for tilt"=w514, "Target for focus"=w514) -> (w568:T6)
                              n180 = call "DataHaso ctor copie.vi"("error in (no error)"=w564, "DataHaso"=w533) -> ("error out"=w567:errorcluster, "new DataHaso"=w566:T4, "DataHaso (dup)"=w532:T4)  [unwired: 3 in]
                              n181 = call "Casao Compute target.vi"("error in (no error)"=w567, "Targets"=w568, "DataHaso"=w566, "Casao"=w557) -> ("error out"=w562:errorcluster, "DataHaso (dup)"=w536:T4, "Casao (dup)"=w563:T10)  [unwired: 1 out]
                              n182 = Bundle By Name(cluster=T5 {"Measurement"=0, "Target"=0, "Manual target"=0} ("Slopes"), "Measurement"=w532, "Target"=w536) -> (w561:T5)
                              n183 = call "Casao get correction commands.vi"("Casao"=w563, "Slopes"=w561, "error in (no error)"=w562) -> ("Casao (dup)"=w535:T10, "Commands"=w528:sgl[], "error out"=w508:errorcluster)  [unwired: 2 in, 2 out]
                              n184 = case shown="True" w511 {
                                tunnel: w508 -> [_ w575]
                                tunnel: w528 -> [_ w574]
                                tunnel: w515 -> [_ w573]
                                frame False {
                                }
                                frame True {
                                n185 = call "PhaseModul apply command.vi"("error in (no error)"=w575, "Commands in"=w574, "Mirror"=w573) -> ()  [unwired: 2 in, 3 out]
                                }
                              }
                            }
                            frame #4 {
                              n186 = call "DataHaso dtor.vi"("Data Haso"=w584) -> ()  [unwired: 6 in, 1 out]
                              n187 = case shown="Error" w578 {
                                tunnel: w577 -> [w585 _]
                                tunnel: [w585 w586] -> w576
                                frame No Error {
                                }
                                frame Error {
                                n188 = Initialize Array(0.0 ("element"), 52 ("dimension size")) -> (w586:dbl[])
                                }
                              }
                            }
                          }
                        }
                      }
                      frame #4 {
                        n189 = call "DataHaso dtor.vi"("Data Haso"=w594) -> ()  [unwired: 6 in, 1 out]
                        n190 = local read "Slice now"() -> (w599:dbl)
                        n191 = Cluster To Array(cluster=w605) -> (array=w604:sgl[])
                        n192 = Build Array (concatenate)(w606, w607, w604, w596) -> (w612:dbl[])
                        n193 = Number To Decimal String(number=w599) -> (decimal integer string=w609:string)  [unwired: 1 in]
                        n194 = Number To Decimal String(number=w599) -> (decimal integer string=w601:string)  [unwired: 1 in]
                        n195 = call "AO single value.vi"("data"=0.0, "physical channels"=tag "Dev1/ao4") -> ()  [unwired: 1 in, 1 out]
                        n196 = call "AO single value.vi"("data"=-5.0, "physical channels"=tag "Dev1/ao5") -> ()  [unwired: 1 in, 1 out]
                        n197 = local read "output path"() -> (w593:path)
                        n198 = Concatenate Strings("afterC_slice", w609, ".dat") -> (w592:string)
                        n199 = Concatenate Strings("command", w601, ".dat") -> (w590:string)
                        n200 = Build Path(base path=w593, name or relative path=w592) -> (appended path=w591:path)
                        n201 = Build Path(base path=w593, name or relative path=w590) -> (appended path=w589:path)
                        n202 = call-poly <vilib>:"Write To Spreadsheet File.vi"("transpose? (no:F)"=TRUE, "format (%.3f)"="%.6f", "1D data"=w612, "file path (dialog if empty)"=w591) -> ()  [unwired: 4 in, 1 out]
                        n203 = call-poly <vilib>:"Write To Spreadsheet File.vi"("transpose? (no:F)"=TRUE, "format (%.3f)"="%.6f", "1D data"=w595, "file path (dialog if empty)"=w589) -> ()  [unwired: 4 in, 1 out]
                      }
                      frame #5 {
                        n204 = local read "Average Frame #"() -> (w619:dbl)
                        n205 = for {
                          N: w619 -> [_]
                          n206 = local read "stop"() -> (w620:bool)
                          n207 = Not(x=w620) -> (.not. x?=w621:bool)
                          n208 = case shown="True" w621 {
                            frame False {
                            }
                            frame True {
                              n209 = flat-sequence {
                                frame #0 {
                                n210 = local read "Laser Power%(0-100)"() -> (w623:dbl)
                                n211 = local read "ImExp Time (s)"() -> (w624:dbl)
                                n212 = local read "Scale factor"() -> (w622:dbl)
                                n213 = call "waveform gen_scale factor.vi"("Scale factor"=w622, "Boolean"=TRUE, "Exposure Time (s)"=w624, "Laser Power%(0-100)"=w623) -> ("waveform"=w626:waveform(dbl)[])
                                n214 = Index Array(array=w626, index=4) -> (element=w634:waveform(dbl))
                                n215 = call "AO triggle.vi"("physical channels"=tag "Dev1/ao0:4", "data"=w626, "waveform"=w634, "trig source"=tag "/Dev1/PFI0") -> ("task out"=w631:refnum<k21>, "error out"=w628:errorcluster)  [unwired: 1 in]
                                n216 = call "DO single value.vi"("error in"=w628, "data"=TRUE, "lines"=tag "Dev1/port0/line0") -> ("error out"=w627:errorcluster)
                                n217 = while {
                                tunnel: [w642] -> w637
                                tunnel: [w641] -> w636
                                tunnel: w631 -> [w639]
                                tunnel: w627 -> [w638]
                                stop <- w640 stop-if-true
                                n218 = call <vilib>:"DAQmx Is Task Done.vi"("task/channels in"=w639, "error in"=w638) -> ("task out"=w642:refnum<k21>, "task done?"=w640:bool, "error out"=w641:errorcluster)  [unwired: 11 in]
                                }
                                n219 = call <vilib>:"DAQmx Clear Task.vi"("task in"=w637, "error in"=w636) -> ()  [unwired: 13 in, 1 out]
                                }
                                frame #1 {
                                n220 = call "AO single value.vi"("data"=0.0, "physical channels"=tag "Dev1/ao4") -> ()  [unwired: 1 in, 1 out]
                                n221 = call "DO single value.vi"("data"=FALSE, "lines"=tag "Dev1/port0/line0") -> ()  [unwired: 1 in, 1 out]
                                }
                              }
                            }
                          }
                        }
                      }
                      frame #6 {
                        n222 = local read "Step size(um)"() -> (w653:dbl)
                        n223 = Multiply(x=w653, y=10.0) -> (x*y=w651:dbl)
                        n224 = Number To Decimal String(number=w651) -> (decimal integer string=w648:string)  [unwired: 1 in]
                        n225 = Concatenate Strings("movrel z=", w648) -> (w649:string)
                        n226 = call "WriteCmd.vi"("Command"=w649, "VISA resource name"=refnum<visa-resource-name> "COM1") -> ()  [unwired: 1 in, 1 out]
                      }
                      frame #7 {
                        n227 = Wait (ms)(milliseconds to wait=u32 50) -> ()  [unwired: 1 out]
                      }
                    }
                  }
                }
                n228 = call "AO single value.vi"("data"=0.0, "physical channels"=tag "Dev1/ao4") -> ()  [unwired: 1 in, 1 out]
              }
            }
            frame #2 {
              n229 = call "Casao dtor.vi"("Casao"=w655) -> ()  [unwired: 6 in, 1 out]
            }
          }
        }
      }
    }
    frame #2 {
      n230 = local read "Step size(um)"() -> (w663:dbl)
      n231 = local read "Slices #"() -> (w656:dbl)
      n232 = Multiply(x=w663, y=-10.0) -> (x*y=w664:dbl)
      n233 = Multiply(x=w664, y=w656) -> (x*y=w662:dbl)
      n234 = Number To Decimal String(number=w662) -> (decimal integer string=w658:string)  [unwired: 1 in]
      n235 = Concatenate Strings("movrel z=", w658) -> (w659:string)
      n236 = call "AO single value.vi"("data"=0.0, "physical channels"=tag "Dev1/ao4") -> ()  [unwired: 1 in, 1 out]
      n237 = call "WriteCmd.vi"("Command"=w659, "VISA resource name"=refnum<visa-resource-name> "COM1") -> ()  [unwired: 1 in, 1 out]
      n238 = call "DO single value.vi"("data"=FALSE, "lines"=tag "Dev1/port0/line1") -> ()  [unwired: 1 in, 1 out]
      n239 = call "DO single value.vi"("data"=FALSE, "lines"=tag "Dev1/port0/line0") -> ()  [unwired: 1 in, 1 out]
    }
  }
